vi "Support Display Time.vi"(11 "Display Time":dbl) -> (3 "Total Array":string[][](array[string]))   [LabVIEW 2023]
uses:
  Modbus/Modbus.lvlib
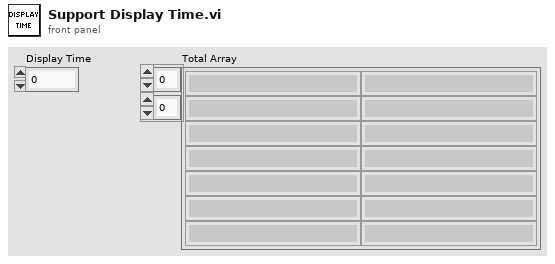
[diagram p1: front panel]
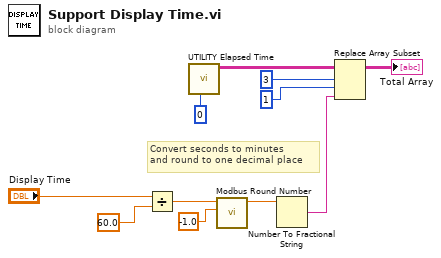
[diagram p0: block diagram]
diagram:
  # "Convert seconds to minutes\nand round to one decimal place"
  n1 = Divide(x="Display Time", y=60.0) -> (x/y=w7:dbl)
  n2 = call "UTILITY Elapsed Time.vi"("precision (6)"=i16 0) -> ("Total Array"=w2:string[][])  [unwired: 6 in, 4 out]
  n3 = call "Modbus Round Number.vi"("Round Decimal Place"=-1.0, "Number"=w7) -> ("Rounded Number"=w8:dbl)  [unwired: 9 in]
  n4 = Number To Fractional String(number=w8) -> (F-format string=w9:string)  [unwired: 3 in]
  n5 = Replace Array Subset(array=w2, new element=w9, index (row)=3 ("disabled index (row)"), index (col)=1 ("disabled index (col)")) -> (→"Total Array":string[][])
